vi "Edit Current Error Code Dialog.vi"(6 "MulticolumnListbox in":refnum<vi>, 8 "Project Path":path, 9 "ItemTag":string, 10 "Error and Descriptions Table":string[][](array[string]), 11 "All Error VIS in":path[](array[path])) -> (3 "All Error VIS out":path[](array[path]))   [LabVIEW 2020, in "ConstantErrorsMaker.lvlib"]
uses:
  ConstantErrorsMaker.lvlib
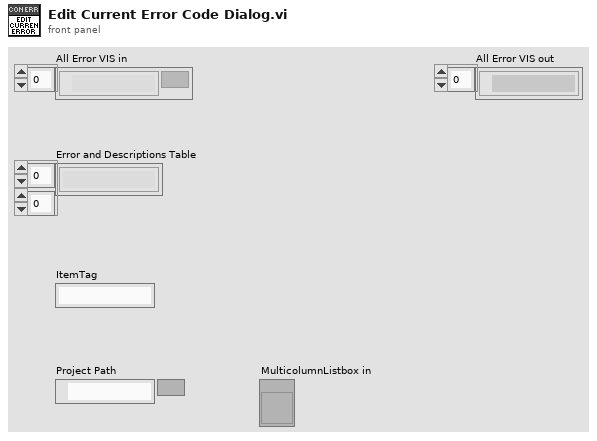
[diagram p1: front panel]
types:
  T1 = typedef "ConstantErrorsMaker.lvlib/MulticolumListbox.ctl" = i32
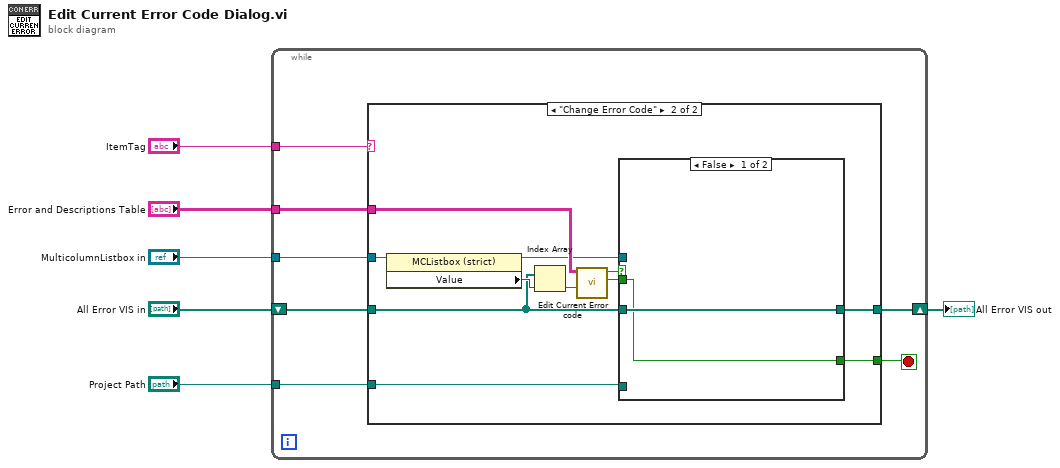
[diagram p0: block diagram]
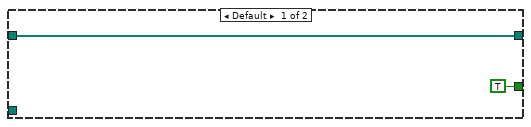
[diagram p2: hidden frame]
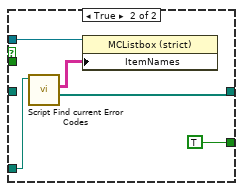
[diagram p3: hidden frame]
diagram:
  n1 = while {
    tunnel: "Project Path" -> [w12]
    tunnel: "Error and Descriptions Table" -> [w11]
    tunnel: "ItemTag" -> [w9]
    tunnel: "MulticolumnListbox in" -> [w8]
    shift-right: [w13] -> w6
    shift-left: "All Error VIS in" -> [w10]
    stop <- w7 stop-if-true
    n2 = case shown="\"Change Error Code\"" w9 {
      tunnel: w10 -> [w15 w20]
      tunnel: w11 -> [_ w24]
      tunnel: w12 -> [_ w23]
      tunnel: [w15 w21] -> w13
      tunnel: w8 -> [_ w19]
      tunnel: [TRUE w17] -> w7
      frame Default {
      }
      frame "Change Error Code" {
        n3 = property class="MCListbox (strict)"(reference=w19) -> (reference out=w18:refnum<vi>, "Value"=w26:T1)  [unwired: 1 in, 1 out]
        n4 = Index Array(array=w20, index=w26) -> (element=w25:path)
        n5 = call "Edit Current Error code.vi"("Error VI Path"=w25, "Error Codes and Descriptions"=w24) -> ("Cancel ?"=w16:bool, "Refresh"=w22:bool)  [unwired: 8 in]
        n6 = case shown="False" w22 {
          tunnel: w23 -> [_ w33]
          tunnel: [w28 w31] -> w21
          tunnel: w20 -> [w28 _]
          tunnel: w18 -> [_ w30]
          tunnel: [w27 TRUE] -> w17
          tunnel: w16 -> [w27 _]
          frame False {
          }
          frame True {
            n7 = call "Script Find current Error Codes.vi"("Selection Owning Folder"=w33) -> ("All Error VIS"=w31:path[], "Error and Descriptions Table"=w32:string[][])  [unwired: 8 in, 1 out]
            n8 = property on="Property Node" class="MCListbox (strict)"(reference=w30, "ItemNames"=w32) -> ()  [unwired: 1 in, 2 out]
          }
        }
      }
    }
  }
  "All Error VIS out" <- w6
